vi "Find Test Cases in LVProj.vi"(8 "error in (no error)":errorcluster, 11 "Project Path":path) -> (0 "error out":errorcluster, 2 "Test Class paths":path[](array[path]))   [LabVIEW 2020, in "Test Finder.lvclass"]
uses:
  Test Finder.lvclass
  API/LUnit Test Case/LUnit Test Case.lvclass
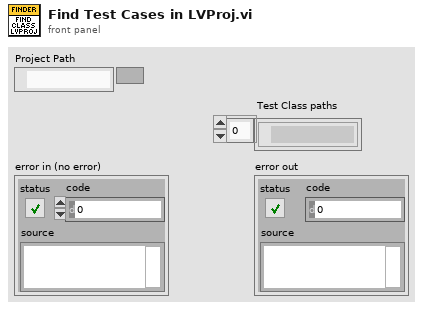
[diagram p1: front panel]
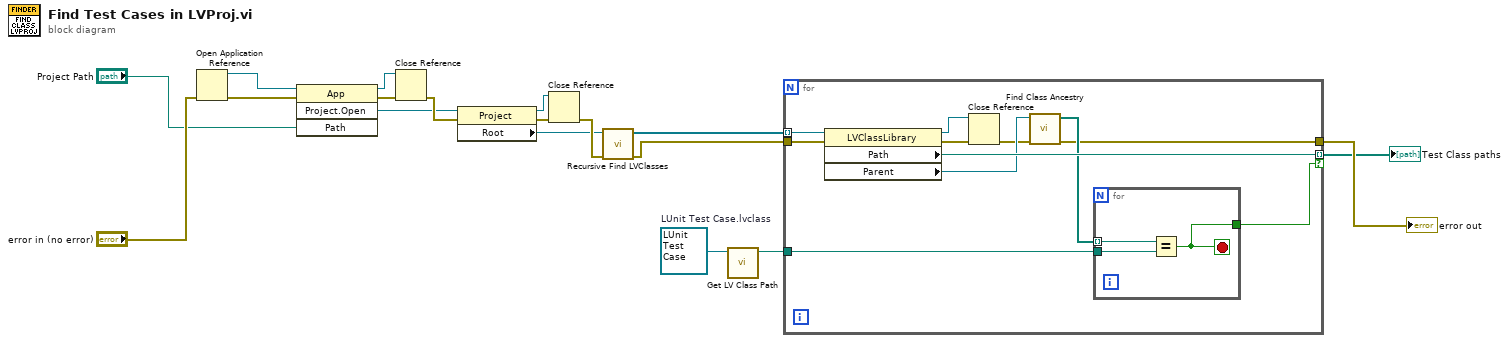
[diagram p0: block diagram]
diagram:
  w2 = refnum<class "LUnit Test Case.lvclass"> refnum  # LUnit Test Case.lvclass
  n1 = Open Application Reference(8:"error in (no error)") -> (0:w8:errorcluster, 3:w7:refnum<vi>)  [unwired: 3 in]
  n2 = invoke class="App" method="Project.Open"(reference=w7, error in=w8, "Path"="Project Path") -> (reference out=w10:refnum<vi>, error out=w9:errorcluster, "Project:Open"=w11:refnum<vi>)  [unwired: 1 in, 1 out]
  n3 = Close Reference(reference=w10, error in (no error)=w9) -> (error out=w12:errorcluster)
  n4 = property class="Project"(reference=w11, error in=w12) -> (reference out=w18:refnum<vi>, error out=w13:errorcluster, "Root"=w3:refnum<vi>)
  n5 = Close Reference(reference=w18, error in (no error)=w13) -> (error out=w17:errorcluster)
  n6 = call "Recursive Find LVClasses.vi"("error in (no error)"=w17, "reference"=w3) -> ("error out"=w4:errorcluster, "Class References"=w14:refnum<vi>[])  [unwired: 8 in]
  n7 = call <vilib>:"Get LV Class Path.vi"("object"=w2) -> ("class path"=w1:path)  [unwired: 9 in, 1 out]
  n8 = for {
    tunnel: w14 -> [w29] mode=indexing
    tunnel: w4 -> [w28]
    tunnel: [w22] -> w16
    tunnel: [w27] -> w5 mode=indexing if=w25
    tunnel: w1 -> [w26]
    n9 = property class="LVClassLibrary"(reference=w29, error in=w28) -> (reference out=w19:refnum<vi>, error out=w24:errorcluster, "Path"=w27:path, "Parent"=w21:refnum<vi>)
    n10 = Close Reference(reference=w19, error in (no error)=w24) -> (error out=w20:errorcluster)
    n11 = call "Find Class Ancestry.vi"("error in (no error)"=w20, "reference in"=w21) -> ("error out"=w22:errorcluster, "Class Ancestry"=w23:path[])  [unwired: 8 in]
    n12 = for {
      tunnel: w23 -> [w31] mode=indexing
      tunnel: w26 -> [w32]
      tunnel: [w30] -> w25
      stop <- w30 stop-if-true
      n13 = Equal?(x=w31, y=w32) -> (x = y?=w30:bool)
    }
  }
  "error out" <- w16
  "Test Class paths" <- w5
